vi "Hi-Tec_Voltage_calculator.vi"(0 "Stack Flowrate (l/min)":dbl=20.0 format="%.2f", 1 "Density Ratio":string, 2 "Mode":enum16{"Control Hi-Tec", "Check Hi-Tec Demands"}(ring), 5 "Strength (% by volume)":dbl=3.0 min=0.0 max=5.0 format="%.2f", 9 "Release temp (deg C)":dbl=20.0 format="%.2f", 11 "Atmos Pres (mbars)":dbl=1000.0 format="%.2f") -> (4 "Carrier 1 Voltage":dbl format="%.3f", 6 "Carrier 2 Voltage":dbl format="%.2f", 8 "Trace Voltage":dbl format="%.2f", 14 "Flowrates (kg/min)":dbl[](array[numeric]) format="%.2f", 15 "Error Comments":string)   [LabVIEW 2010]
panel:
  # "-Carrier 1 only\n-Carrier 2 only\n-Enter Ratio"
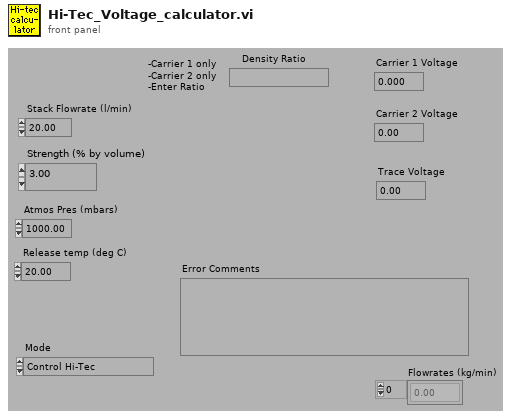
[diagram p1: front panel]
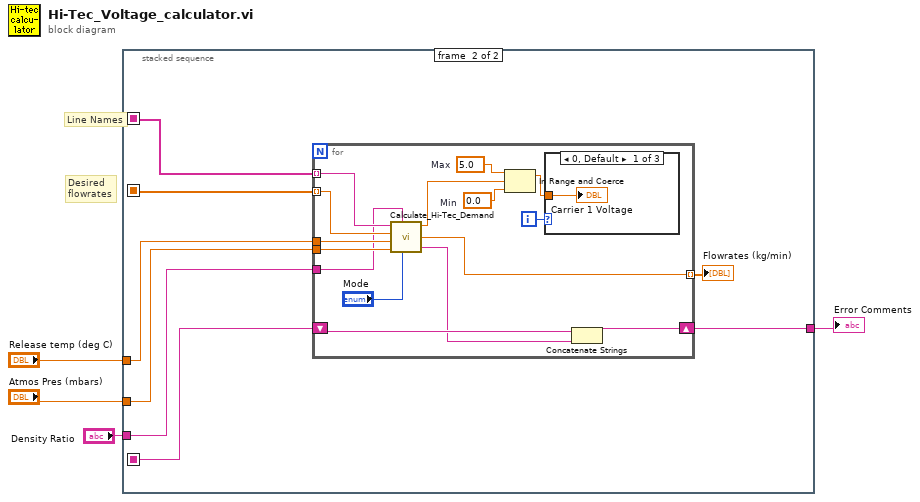
[diagram p0: block diagram]
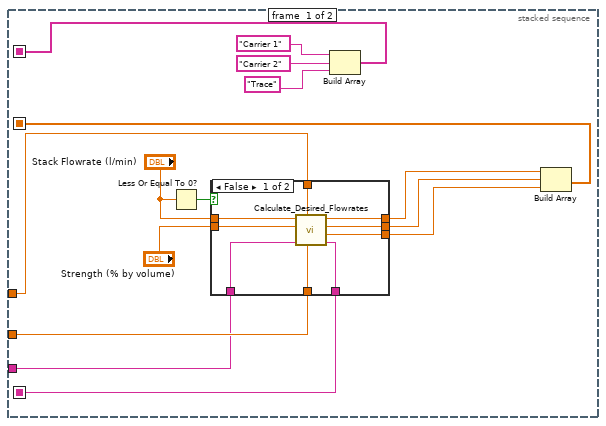
[diagram p2: hidden frame]
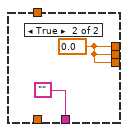
[diagram p3: hidden frame]
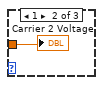
[diagram p4: hidden frame]
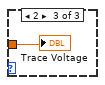
[diagram p5: hidden frame]
diagram:
  # "Line Names"
  # "Desired\nflowrates"
  n1 = stacked-sequence {
    seq-local: [w13 _] -> [_ w36]
    seq-local: [w9 _] -> [_ w35]
    seq-local: [w8 _] -> [_ w31]
    tunnel: "Release temp (deg C)" -> [w18 w37]
    tunnel: "Atmos Pres (mbars)" -> [w17 w38]
    tunnel: "Density Ratio" -> [w7 w33]
    tunnel: [_ w34] -> w1
    frame #0 {
      n2 = Less Or Equal To 0?(x="Stack Flowrate (l/min)") -> (x <= 0?=w5:bool)
      n3 = case shown="False" w5 {
        tunnel: "Stack Flowrate (l/min)" -> [w28 _]
        tunnel: "Strength (% by volume)" -> [w27 _]
        tunnel: w18 -> [w26 _]
        tunnel: w17 -> [w25 _]
        tunnel: [w24 w30] -> w16
        tunnel: [w23 w30] -> w15
        tunnel: [w22 w30] -> w14
        tunnel: [w21 ""] -> w8
        tunnel: w7 -> [w20 _]
        frame False {
          n4 = call "Calculate_Desired_Flowrates.vi"("Atmos Pres (mbars)"=w25, "Release temp (deg C)"=w26, "Density Ratio"=w20, "Strength (% by volume)"=w27, "Stack Flowrate (l/min)"=w28) -> ("Error Message"=w21:string, "Trace Q l/min"=w22:dbl, "Carrier 2 l/min"=w23:dbl, "Carrier 1 l/min"=w24:dbl)  [unwired: 1 out]
        }
        frame True {
          w30 = 0.0 ("Carrier 1 l/min")
        }
      }
      n5 = Build Array("Carrier 1" ("Gas Line Name"), "Carrier 2" ("Gas Line Name"), "Trace" ("Gas Line Name")) -> (w9:string[])
      n6 = Build Array(w16, w15, w14) -> (w13:dbl[])
    }
    frame #1 {
      n7 = for {
        shift-right: [w50] -> w34
        shift-left: w31 -> [w52]
        tunnel: w38 -> [w49]
        tunnel: w37 -> [w48]
        tunnel: w36 -> [w47] mode=indexing
        tunnel: [w40] -> w32 mode=indexing
        tunnel: w35 -> [w46] mode=indexing
        tunnel: w33 -> [w45]
        i -> [w53]
        w42 = 0.0  # Min
        w43 = 5.0  # Max
        n8 = call "Calculate_Hi-Tec_Demand.vi"("Gas Line Name"=w46, "Density Ratio"=w45, "Flowrate"=w47, "Release temp (deg C)"=w48, "Mode"="Mode", "Atmos Pres (mbars)"=w49) -> ("Demand Voltage"=w41:dbl, "Flowrate (kg/min)"=w40:dbl, "Error messages"=w51:string)
        n9 = In Range and Coerce(upper limit=w43, x=w41, lower limit=w42) -> (coerced(x)=w39:dbl)  [unwired: 1 out]
        n10 = case shown="0, Default" w53 {
          tunnel: w39 -> [w54 w55 w56]
          frame 0, Default {
            "Carrier 1 Voltage" <- w54
          }
          frame 1 {
            "Carrier 2 Voltage" <- w55
          }
          frame 2 {
            "Trace Voltage" <- w56
          }
        }
        n11 = Concatenate Strings(w52, w51) -> (w50:string)
      }
      "Flowrates (kg/min)" <- w32
    }
  }
  "Error Comments" <- w1
